vi "Start Form Server.vi"(8 "error in (no error)":errorcluster, 9 "Database":refnum<class "Database Adv Schema.lvclass">, 10 "Custom Form Server":refnum<class "Form Server.lvclass">) -> (0 "error out":errorcluster, 3 "Form Server Wrapper out":refnum<class "Form Server Wrapper.lvclass">)   [LabVIEW 2020, in "Form Server.lvlib" / "Form Server Wrapper.lvclass"]
uses:
  Form Server Wrapper.lvclass
  Form Server/Form Server.lvclass
  C:/Program Files (x86)/National Instruments/LabVIEW 2020/vi.lib/ActorFramework/Actor/Actor.lvclass
  Database OOP/Database Libraries/Database Interfaces/Database Advanced Schema Class/Database Adv Schema.lvclass
  Form Server Wrapper.lvclass/Form Server Wrapper.ctl
  Form Server Configuration/Form Server Configuration.lvclass
  Open Close Logic Simple Table/Open Close Logic Simple Table.lvclass
  C:/Users/User/Desktop/Raman Program/Database OOP/source/Forms AF/Autoclose manager/Open Close Logic.lvclass
  Form Server Configuration/Form Server Configuration.lvclass/Form Server Configuration.ctl
  Form Server/Form Server.lvclass/Form Server.ctl
  <vilib>/ActorFramework/Actor/Actor.lvclass
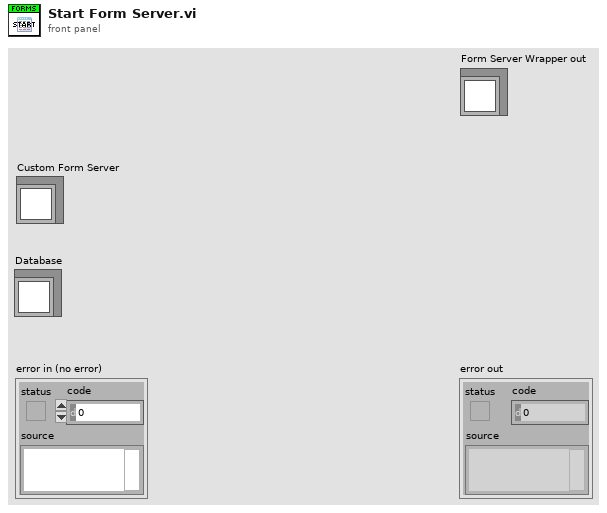
[diagram p1: front panel]
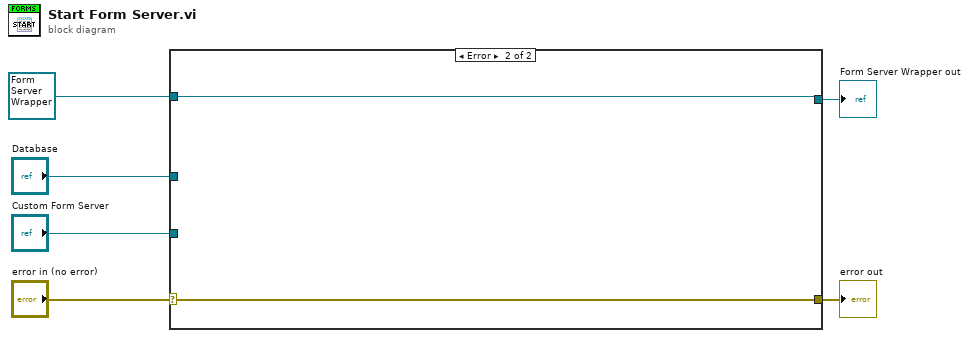
[diagram p0: block diagram]
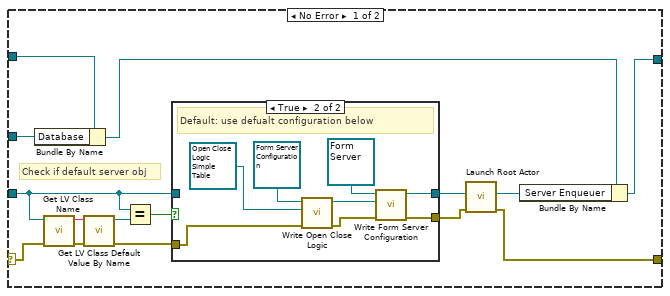
[diagram p2: hidden frame]
diagram:
  n1 = case shown="Error" "error in (no error)" {
    selector: "error in (no error)" -> [w12 w33]
    tunnel: [w14 w33] -> w5
    tunnel: "Custom Form Server" -> [w17 _]
    tunnel: "Database" -> [w9 _]
    tunnel: refnum<class "Form Server Wrapper.lvclass"> refnum ("Form Server Wrapper out") -> [w8 w32]
    tunnel: [w7 w32] -> w1
    frame No Error {
      # "Check if default server obj"
      n2 = Bundle By Name(cluster=w8, "Database"=w9) -> (w10:refnum<class "Form Server Wrapper.lvclass">)
      n3 = call <vilib>:"Get LV Class Name.vi"("error in (no error)"=w12, "object"=w17) -> ("error out"=w21:errorcluster, "class name"=w20:string)  [unwired: 8 in]
      n4 = call <vilib>:"Get LV Class Default Value By Name.vi"("error in (no error)"=w21, "class name"=w20) -> ("error out"=w11:errorcluster, "object"=w19:refnum<class>)  [unwired: 8 in]
      n5 = Equal?(x=w17, y=w19) -> (x = y?=w18:bool)
      n6 = case shown="True" w18 {
        tunnel: w17 -> [w23 _]
        tunnel: [w23 w27] -> w16
        tunnel: w11 -> [w22 w24]
        tunnel: [w22 w25] -> w15
        frame False {
          # "Not default: use as configured"
        }
        frame True {
          # "Default: use defualt configuration below"
          n7 = call "Write Open Close Logic.vi"("error in (no error)"=w24, "Form Server Interfaces.lvlib:Open Close Logic.lvclass"=refnum<class "Open Close Logic Simple Table.lvclass"> refnum ("Open Close Logic Simple Table.lvlib:Open Close Logic Simple Table.lvclass"), "Form Server Configuration in"=refnum<class "Form Server Configuration.lvclass"> refnum ("Form Server Configuration.lvlib:Form Server Configuration.lvclass")) -> ("error out"=w26:errorcluster, "Form Server Configuration out"=w29:refnum<class "Form Server Configuration.lvclass">)  [unwired: 7 in]
          n8 = call "Write Form Server Configuration.vi"("error in (no error)"=w26, "Form Server Configuration.lvlib:Form Server Configuration.lvclass"=w29, "Form Server in"=refnum<class "Form Server.lvclass"> refnum ("Form Server.lvlib:Form Server.lvclass")) -> ("error out"=w25:errorcluster, "Form Server out"=w27:refnum<class "Form Server.lvclass">)  [unwired: 7 in]
        }
      }
      n9 = call <vilib>:"Launch Root Actor.vi"("error in (no error)"=w15, "Actor"=w16) -> ("error out"=w14:errorcluster, "Actor's Enqueuer"=w13:refnum<class "Message Enqueuer.lvclass">)  [unwired: 8 in]
      n10 = Bundle By Name(cluster=w10, "Server Enqueuer"=w13) -> (w7:refnum<class "Form Server Wrapper.lvclass">)
    }
    frame Error {
    }
  }
  "error out" <- w5
  "Form Server Wrapper out" <- w1
